vi "UMLEditor reversedEngineeringRecursiveSetPos.vi"(0 "BlockXpos":i32, 1 "startYpos":i32, 2 "nodeIndex":i32, 3 "widthGap":i32=50, 4 "heightGap":i32=50, 5 "error in (no error)":errorcluster, 6 "localIn":T1 {"block"."bounds"."height" format="%.2f"; "block"."bounds"."width" format="%.2f"; "block"."bounds"."y" format="%.2f"; "block"."bounds"."x" format="%.2f"; "bounds"."height" format="%.2f"; "bounds"."width" format="%.2f"; "bounds"."y" format="%.2f"; "bounds"."x" format="%.2f"}) -> (12 "localOut":T1 {"block"."bounds"."height" format="%.2f"; "block"."bounds"."width" format="%.2f"; "block"."bounds"."y" format="%.2f"; "block"."bounds"."x" format="%.2f"; "bounds"."height" format="%.2f"; "bounds"."width" format="%.2f"; "bounds"."y" format="%.2f"; "bounds"."x" format="%.2f"}, 19 "error out":errorcluster)   [LabVIEW 2012]
doc: "Gets current diagram values"
uses:
  <resource>/Framework/Providers/Open_GDS/UML/UMLEditor/UMLEditor RevEngLocalvarType.ctl
  <resource>/Framework/Providers/Open_GDS/UML/Graph_class/Graph.lvclass
  <resource>/Framework/Providers/Open_GDS/UML/Graphics_class/Graphics.lvclass
  <resource>/Framework/Providers/Open_GDS/UML/Grid_class/Grid.lvclass
  <resource>/Framework/Providers/Open_GDS/UML/ClassNode_class/ClassNode.lvclass
  <resource>/Framework/Providers/Open_GDS/UML/AbstractEdge_class/AbstractEdge.lvclass
  <resource>/Framework/Providers/Open_GDS/UML/AbstractNode_class/AbstractNode.lvclass
  <resource>/Framework/Providers/Open_GDS/UML/ReversedEngineering/ReversedEngineering ClassInfoType.ctl
  <resource>/Framework/Providers/Open_GDS/UML/UMLEditor/UMLEditor_VisibilityType.ctl
  <resource>/Framework/Providers/Open_GDS/UML/ReversedEngineering/ReversedEngineering AttributeInfoType.ctl
  <resource>/Framework/Providers/Open_GDS/ClassProviders/Common/CommonVIs/CommonVIs_AttributeDataType.ctl
  <resource>/Framework/Providers/Open_GDS/UML/ReversedEngineering/ReversedEngineering_ClassDependencyDetailsType.ctl
  <resource>/Framework/Providers/Open_GDS/ClassProviders/Common/ScriptingFunctions/SubVIs/Scripting_ViDependencyType.ctl
  <resource>/Framework/Providers/Open_GDS/UML/General/Rectangle/Rectangle Rectangle2D.ctl
  <resource>/Framework/Providers/Open_GDS/UML/ReversedEngineering/ReversedEngineering TypeDefType.ctl
panel:
  in  "type specifier VI Refnum (for type only)":refnum<vi>
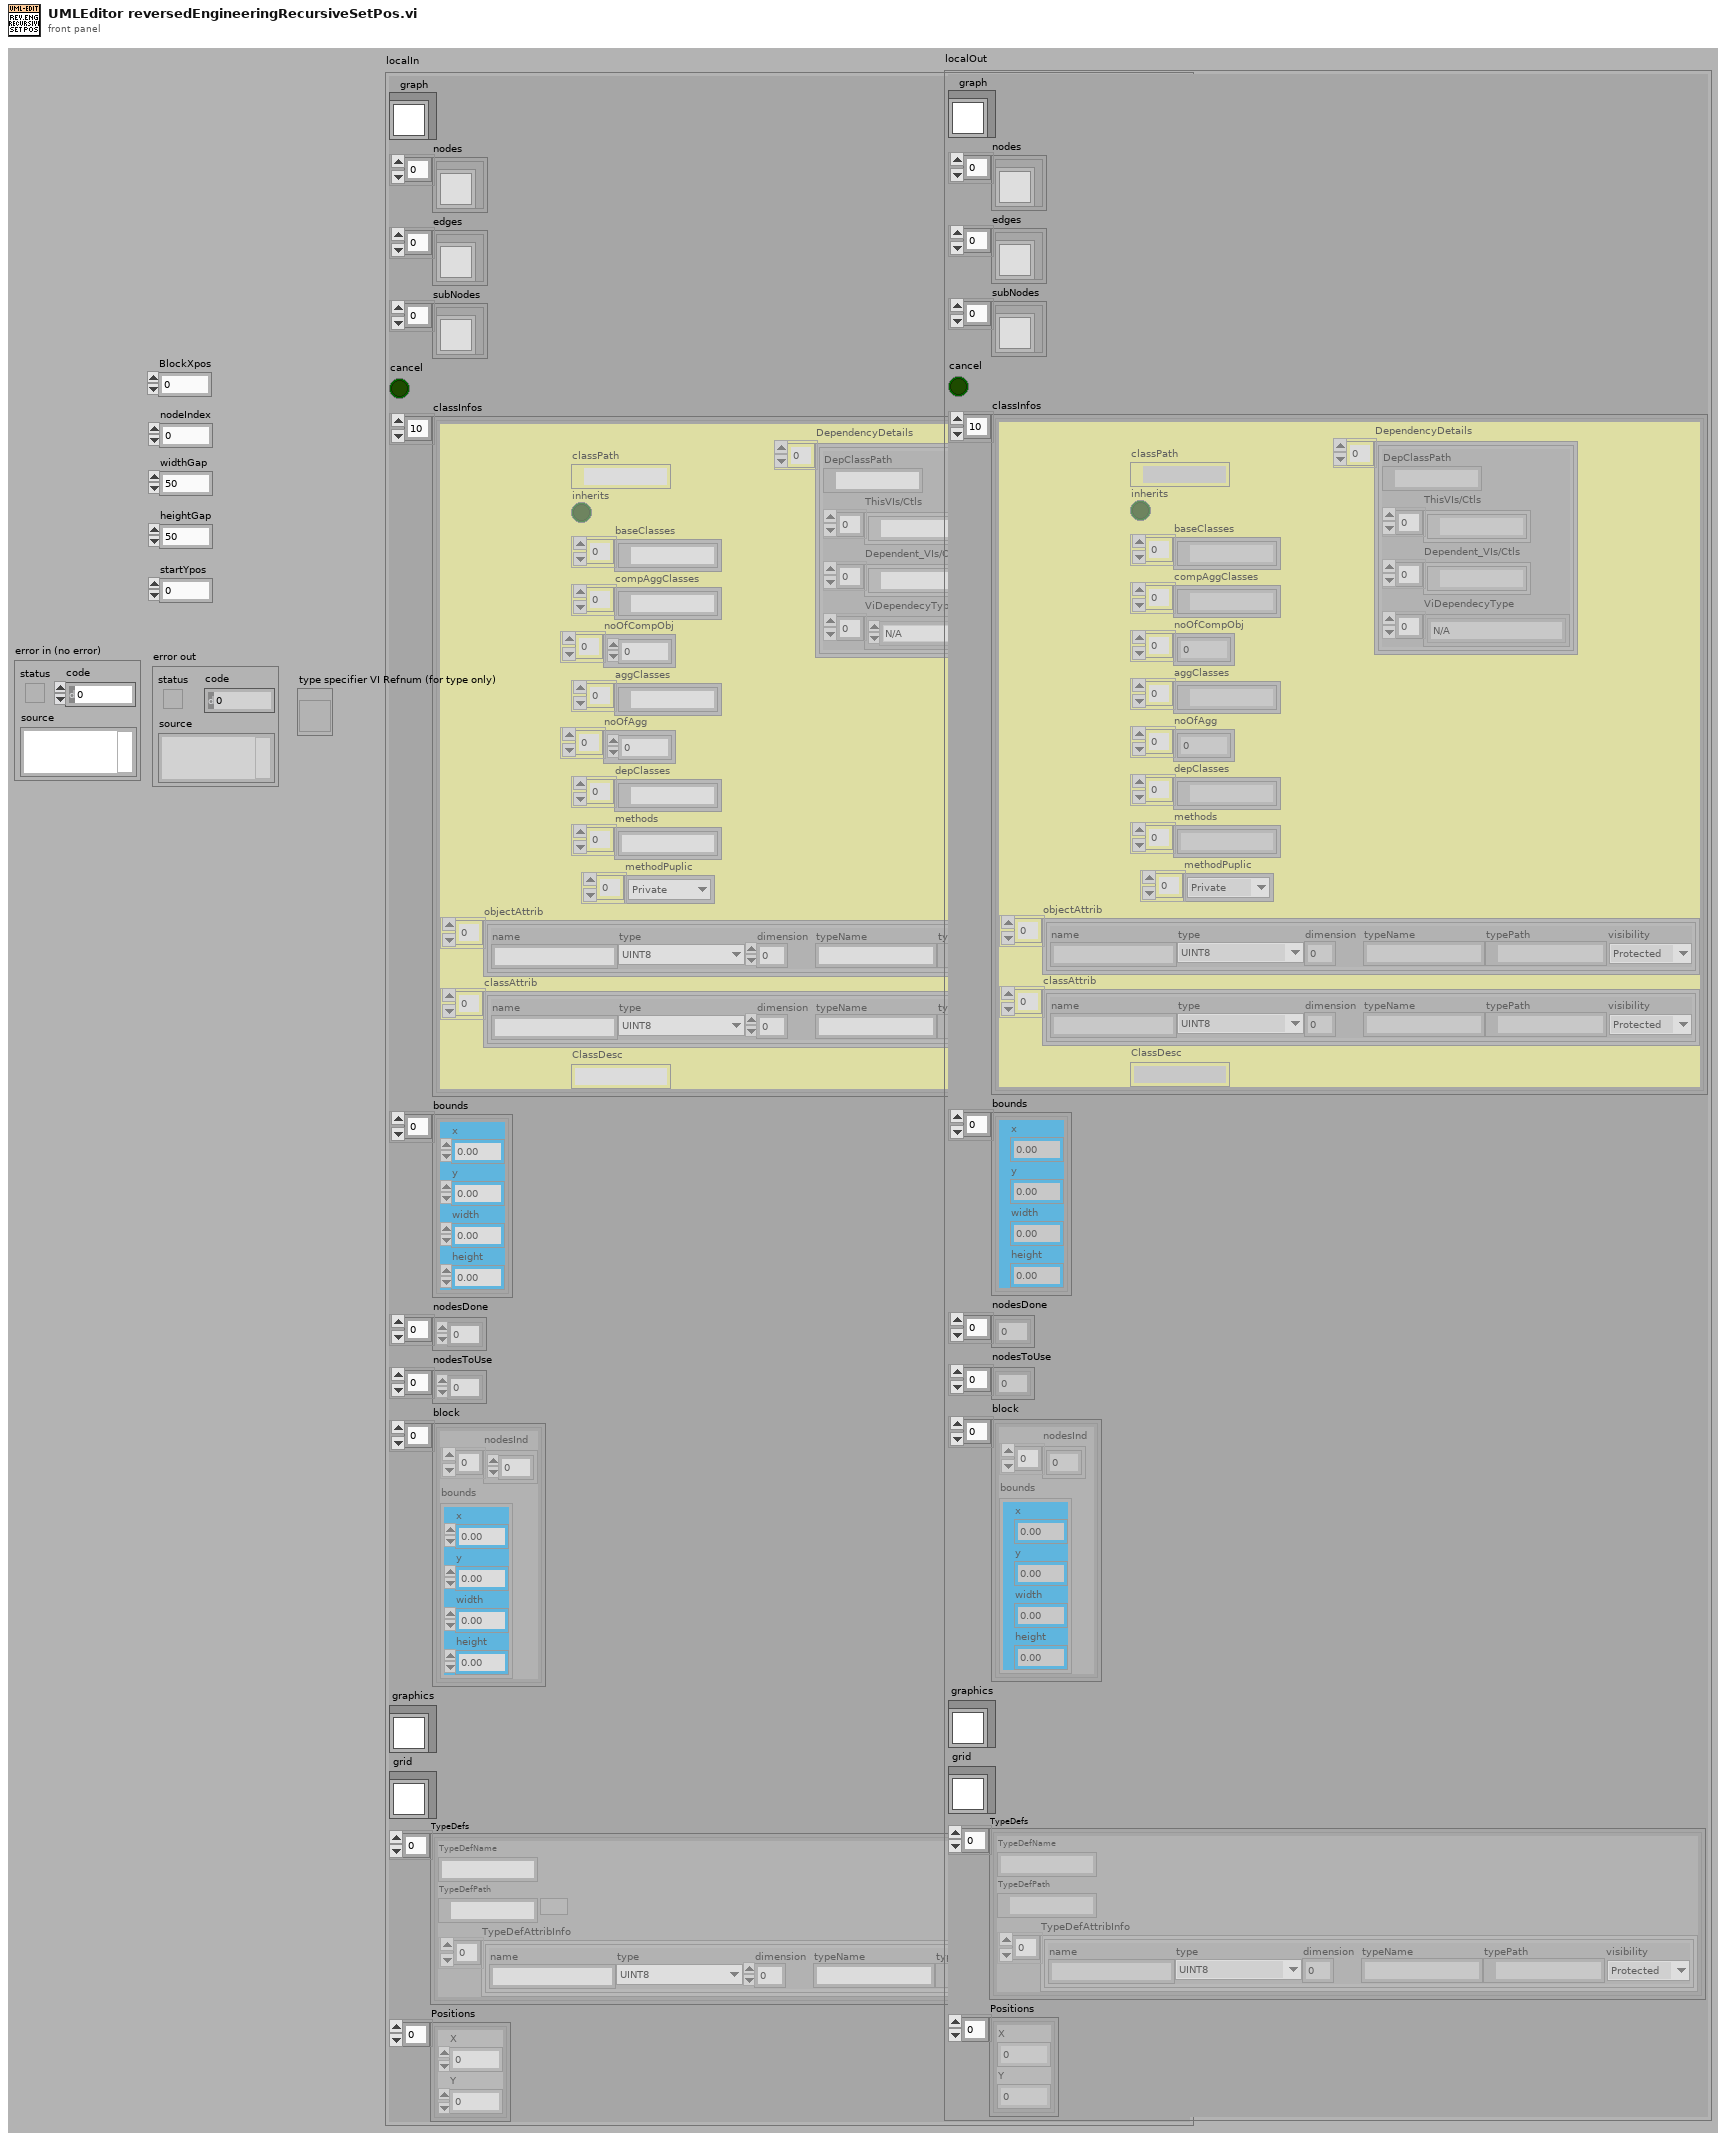
[diagram p1: front panel]
types:
  T1 = typedef "UMLEditor RevEngLocalvarType.ctl" = cluster{"graph":refnum<class "Graph.lvclass">, "nodes":refnum<class "ClassNode.lvclass">[], "edges":refnum<class "AbstractEdge.lvclass">[], "subNodes":refnum<class "AbstractNode.lvclass">[], "cancel":bool, "classInfos":T2[], "bounds":T8[], "nodesDone":i32[], "nodesToUse":i32[], "block":cluster{"nodesInd":i32[], "bounds":T8}[], "graphics":refnum<class "Graphics.lvclass">, "grid":refnum<class "Grid.lvclass">, "TypeDefs":T9[], "Positions":cluster{"X":i32, "Y":i32}[]}
  T2 = typedef "ReversedEngineering ClassInfoType.ctl" = cluster{"classPath":path, "inherits":bool, "baseClasses":path[], "compAggClasses":path[], "noOfCompObj":i32[], "aggClasses":path[], "noOfAgg":i32[], "depClasses":path[], "methods":string[], "methodPuplic":T3[], "objectAttrib":T4[], "classAttrib":T4[], "ClassDesc":string, "DependencyDetails":T6[]}
  T3 = typedef "UMLEditor_VisibilityType.ctl" = enum16{"Public", "Private", "Protected"}
  T4 = typedef "ReversedEngineering AttributeInfoType.ctl" = cluster{"name":string, "type":T5, "dimension":i32, "typeName":string, "typePath":path, "visibility":T3}
  T5 = typedef "CommonVIs_AttributeDataType.ctl" = enum16{"UINT8", "INT8", "UINT16", "INT16", "UINT32", "INT32", "UINT64", "INT64", "SGL", "DBL", "EXT", "CSG", "CDB", "CXT", "TimeStamp", "STRING", "PATH", "BOOL", "ENUM", "RefNum", "VIRefNum", "LabVIEW Class", "Cluster", "Variant", "TypeDef", "Waveform", "LabVIEW Object", "Other", "void"}
  T6 = typedef "ReversedEngineering_ClassDependencyDetailsType.ctl" = cluster{"DepClassPath":path, "ThisVIs/Ctls":path[], "Dependent_VIs/Ctls":path[], "ViDependecyType":T7[]}
  T7 = typedef "Scripting_ViDependencyType.ctl" = enum16{"N/A", "Launches"}
  T8 = typedef "Rectangle Rectangle2D.ctl" = cluster{"x":dbl, "y":dbl, "width":dbl, "height":dbl}
  T9 = typedef "ReversedEngineering TypeDefType.ctl" = cluster{"TypeDefName":string, "TypeDefPath":path, "TypeDefAttribInfo":T4[]}
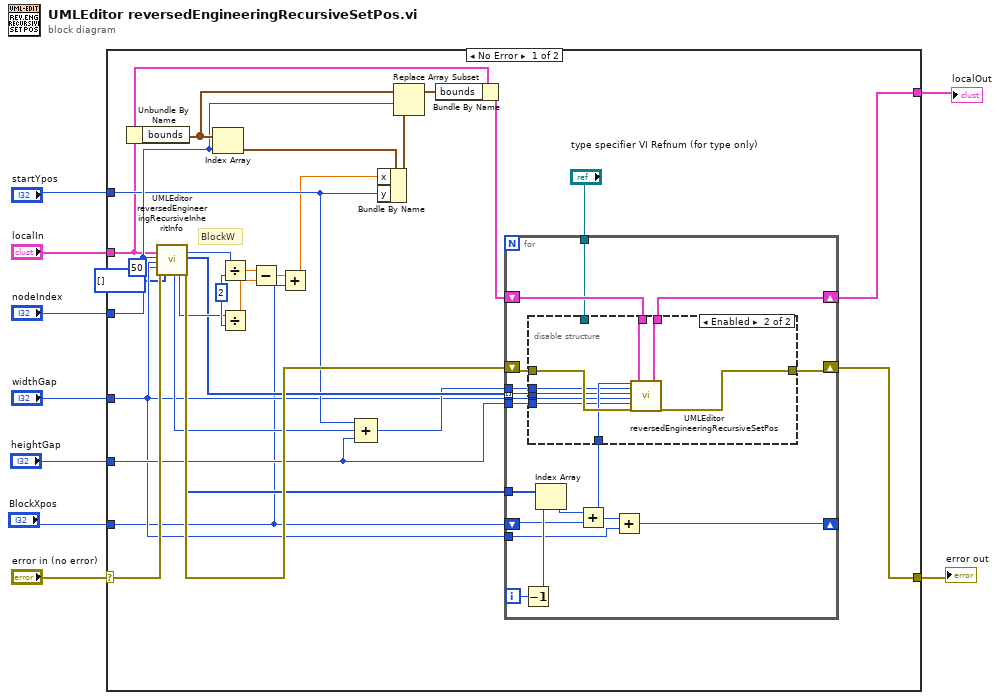
[diagram p0: block diagram]
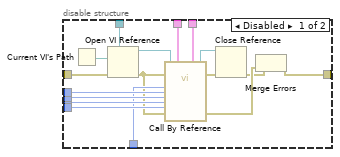
[diagram p2: hidden frame]
diagram:
  n1 = case shown="No Error" "error in (no error)" {
    selector: "error in (no error)" -> [w36 w83]
    tunnel: [w38 w83] -> w8
    tunnel: "localIn" -> [w19 w82]
    tunnel: "nodeIndex" -> [w27 _]
    tunnel: "widthGap" -> [w15 _]
    tunnel: [w17 w82] -> w4
    tunnel: "startYpos" -> [w23 _]
    tunnel: "heightGap" -> [w20 _]
    tunnel: "BlockXpos" -> [w14 _]
    frame No Error {
      w34 = 2 ("y")
      # "BlockW"
      n2 = Unbundle By Name(w19) -> ("bounds"=w28:T8[])
      n3 = call <resource>:"UMLEditor reversedEngineeringRecursiveInheritInfo.vi"("localIn"=w19, "nodeIndex"=w27, "widthGap"=w15, "heightGap"=50, "error in (no error)"=w36, "allInheritorIn"=i32[] []) -> ("myHeight"=w22:i32, "myWidth"=w32:i32, "width"=w35:i32, "myInheritor"=w25:i32[], "myInheritorWidth"=w16:i32[], "error out"=w37:errorcluster)  [unwired: 8 out]
      n4 = Index Array(array=w28, index=w27) -> (element=w30:T8)
      n5 = Divide(x=w35, y=w34) -> (x/y=w33:dbl)
      n6 = Divide(x=w32, y=w34) -> (x/y=w31:dbl)
      n7 = Subtract(x=w33, y=w31) -> (x-y=w13:dbl)
      n8 = Add(x=w13, y=w14) -> (x+y=w12:dbl)
      n9 = Compound Arithmetic op=ADD(w23, w22, w20) -> (w21:i32)
      n10 = Bundle By Name(cluster=w30, "x"=w12, "y"=w23) -> (w26:T8)
      n11 = Replace Array Subset(array=w28, new element=w26, index=w27) -> (w29:T8[])
      n12 = Bundle By Name(cluster=w19, "bounds"=w29) -> (w18:T1)
      n13 = for {
        tunnel: w15 -> [w55]
        shift-right: [w49] -> w38
        shift-left: w37 -> [w54]
        tunnel: w25 -> [w53] mode=indexing
        shift-right: [w51] -> w17
        shift-left: w18 -> [w52]
        tunnel: "type specifier VI Refnum (for type only)" -> [w50]
        tunnel: w21 -> [w48]
        tunnel: w20 -> [w47]
        tunnel: w16 -> [w46]
        shift-right: [w39] -> _
        shift-left: w14 -> [w43]
        tunnel: w15 -> [w40]
        i -> [w45]
        n14 = Decrement(x=w45) -> (x-1=w44:i32)
        n15 = Index Array(array=w46, index=w44) -> (element=w42:i32)
        n16 = Add(x=w42, y=w43) -> (x+y=w41:i32)
        n17 = disable-structure shown="Enabled" {
          disable-tunnel: w55 -> [w68 w75]
          disable-tunnel: w54 -> [w67 w79]
          disable-tunnel: w53 -> [w66 w74]
          disable-tunnel: w52 -> [w65 w81]
          disable-tunnel: [w64 w80] -> w51
          disable-tunnel: w50 -> [w63 _]
          disable-tunnel: [w60 w78] -> w49
          disable-tunnel: w48 -> [w59 w76]
          disable-tunnel: w47 -> [w58 w73]
          disable-tunnel: w41 -> [w57 w77]
          frame Disabled {
            n18 = Current VI's Path() -> (path=w72:path)
            n19 = Open VI Reference(type specifier VI Refnum (for type only)=w63, vi path=w72, error in (no error)=w67) -> (vi reference=w71:refnum<vi>, error out=w56:errorcluster)  [unwired: 3 out]
            n20 = call-by-ref "?"(reference=w71, error in=w56, "BlockXpos"=w57, "startYpos"=w59, "nodeIndex"=w66, "widthGap"=w68, "heightGap"=w58, "error in (no error)"=w56, "localIn"=w65) -> (reference out=w70:refnum<vi>, error out=w69:errorcluster, "localOut"=w64:T1, 19:"error out"=w62:errorcluster)  [unwired: 11 in]
            n21 = Close Reference(reference=w70, error in (no error)=w69) -> (error out=w61:errorcluster)
            n22 = Merge Errors(w61, w62) -> (w60:errorcluster)
          }
          frame Enabled {
            n23 = call <resource>:"UMLEditor reversedEngineeringRecursiveSetPos.vi"("BlockXpos"=w77, "startYpos"=w76, "nodeIndex"=w74, "widthGap"=w75, "heightGap"=w73, "error in (no error)"=w79, "localIn"=w81) -> ("localOut"=w80:T1, "error out"=w78:errorcluster)  [unwired: 11 in]
          }
        }
        n24 = Add(x=w41, y=w40) -> (x+y=w39:i32)
      }
    }
    frame Error {
    }
  }
  "error out" <- w8
  "localOut" <- w4
